vi "Actor Core.vi"(8 "error in":errorcluster, 11 "SimpleChart In":refnum<class "SimpleChart.lvclass">) -> (0 "error out":errorcluster, 3 "Actor out":refnum<class "Actor.lvclass">)   [LabVIEW 2015, in "MVAExamples.lvlib" / "SimpleChart.lvclass"]
doc: "(<B>Filename</B>: Actor Framework.lvlib:Actor.lvclass:Actor Core.vi)\n\nReceives messages to the actor, reacts to them, and initiates any error handling that may shut the actor down.\n\nDescendant classes may override this VI to append parallel tasks for the actor to complete while it handles messages. Overrides use the Call Parent Method node.\n\n<License>\nCopyright © 2017 Composed Systems, LLC | All rights reserved\nwww.composed.io\n\nAuthor: Ethan Stern <ethan.stern@composed.io>\n\nThis software is provided \"AS IS\" WITHOUT WARRANTIES, either express or implied, AND IS FOR EDUCATIONAL PURPOSES ONLY.\n</License>"
uses:
  SimpleChart.lvclass
  <vilib>/ActorFramework/Actor/Actor.lvclass
  SimpleChart.lvclass/SimpleChart.ctl
  Framework/IViewable/IViewable/IViewable.lvclass
panel:
  out "Simulated Data":dbl(graph)
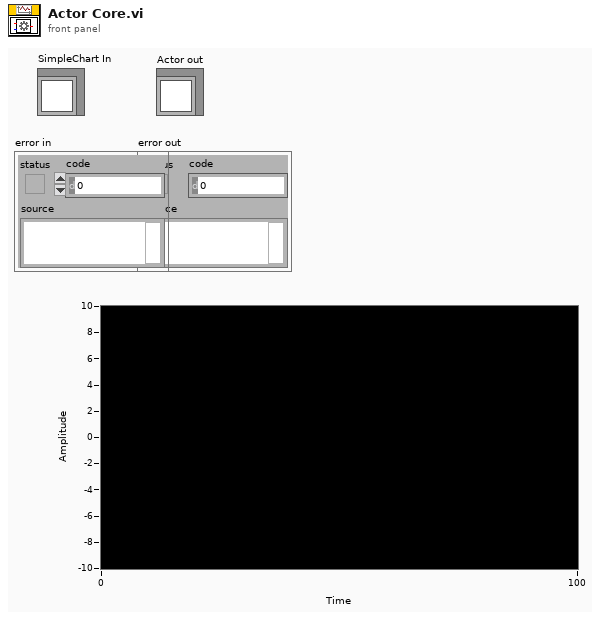
[diagram p1: front panel]
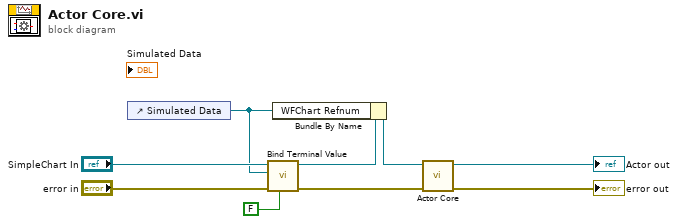
[diagram p0: block diagram]
diagram:
  n1 = control-ref of="Simulated Data"() -> (w1:refnum<vi>)
  n2 = call "Bind Terminal Value.vi"("Value Changes Only? (T)"=FALSE, "error in (no error)"="error in", "Ctl Refnum"=w1, "IViewable in"="SimpleChart In") -> ("error out"=w4:errorcluster, "IViewable out"=w6:refnum<class "SimpleChart.lvclass">)  [unwired: 6 in]
  n3 = Bundle By Name(cluster=w6, "WFChart Refnum"=w1) -> (w2:refnum<class "SimpleChart.lvclass">)
  n4 = call-parent "Actor Core.vi"("error in"=w4, "IViewable In"=w2) -> ("error out"=→"error out":errorcluster, "Actor out"=→"Actor out":refnum<class "Actor.lvclass">)  [unwired: 8 in]
